vi "例程42-局部变量.vi"() -> ()   [LabVIEW 2016]
panel:
  in  "停止":bool
  out "波形图表 3":dbl(graph)
  out "波形图表":dbl(graph)
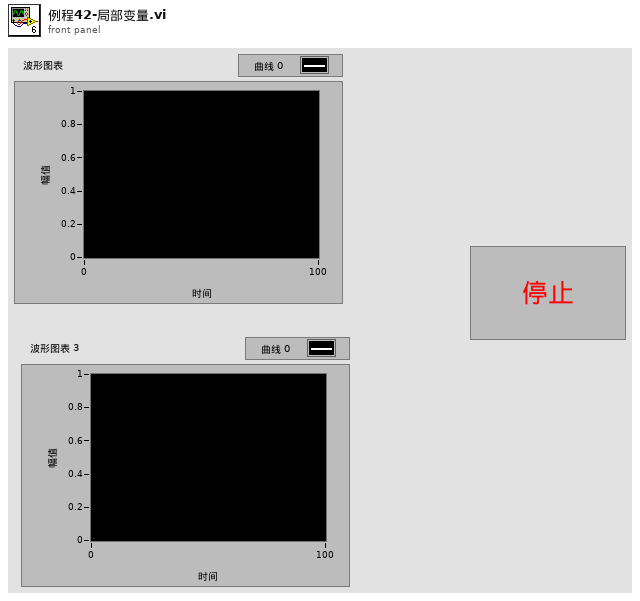
[diagram p1: front panel]
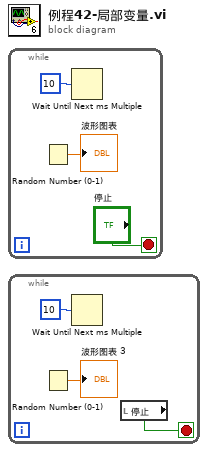
[diagram p0: block diagram]
diagram:
  n1 = while {
    stop <- "停止" stop-if-true
    n2 = Random Number (0-1)() -> (number: 0 to 1=→"波形图表":dbl)
    n3 = Wait Until Next ms Multiple(millisecond multiple=u32 10 ("毫秒倍数")) -> ()  [unwired: 1 out]
  }
  n4 = while {
    stop <- w4 stop-if-true
    n5 = Random Number (0-1)() -> (number: 0 to 1=→"波形图表 3":dbl)
    n6 = Wait Until Next ms Multiple(millisecond multiple=u32 10 ("毫秒倍数")) -> ()  [unwired: 1 out]
    n7 = local read "停止"() -> (w4:bool)
  }
